vi "Drive Action.vi"(8 "Motor Saftey":T1, 11 "Operation States":T3) -> ()   [LabVIEW 2014]
uses:
  <vilib>/Rock Robotics/WPI/Solenoid/WPI_SolenoidValue.ctl
  <vilib>/Rock Robotics/WPI/SafetyOutput/WPI_SafetyOutputConfigMenu.ctl
  <vilib>/Rock Robotics/WPI/RobotDrive/WPI_RobotDriveGetSetRefNum.vi
  Robot Global Data.vi
  <vilib>/Rock Robotics/Network Tables/SD Write Numeric Array.vi
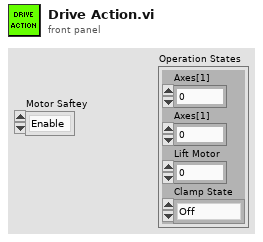
[diagram p1: front panel]
types:
  T1 = typedef "WPI_SafetyOutputConfigMenu.ctl" = enum16{"Enable", "Disable"}
  T2 = typedef "WPI_SolenoidValue.ctl" = enum16{"Off", "On", "Forward", "Reverse"}
  T3 = cluster{"Axes[1]":dbl, "Axes[1]":dbl, "Lift Motor":dbl, "Clamp State":T2}
  T4 = typedef "WPI_RobotDriveDevRef.ctl" = cluster{"DevStatus":errorcluster, "Motors[]":T5[], "Square Inputs":bool, "Max Output":dbl}
  T5 = typedef "WPI_MotorControlDeviceRef.ctl" = cluster{"DeviceStatus":errorcluster, "Type":T6, "PWM":cluster{"Controller":T7, "PWM Channel":T8, "DeadBand":T9}, "CAN":cluster{"Device Number":u8, "Control Mode":T10, "Semaphore":T11, "Max Vout":dbl, "TalonSRX Control Mode":T12}, "Invert":bool, "TransformRef":T13, "InvTransformRef":T13}
  T6 = typedef "WPI_MotorControlType.ctl" = enum16{"PWM", "CAN", "CANTalonSRX"}
  T7 = typedef "FPGA_TypedefDigitalModule.ctl" = enum16{"Controller 1"}
  T8 = typedef "FPGA_DIOPWMChannel.ctl" = enum8{"PWM 0", "PWM 1", "PWM 2", "PWM 3", "PWM 4", "PWM 5", "PWM 6", "PWM 7", "PWM 8", "PWM 9", "PWM MXP 0", "PWM MXP 1", "PWM MXP 2", "PWM MXP 3", "PWM MXP 4", "PWM MXP 5", "PWM MXP 6", "PWM MXP 7", "PWM MXP 8", "PWM MXP 9", "Invalid"}
  T9 = typedef "WPI_PWMDeadband.ctl" = cluster{"Name":string, "maxPositivePwm":i32, "minPositivePwm":i32, "centerPwm":i32, "maxNegativePwm":i32, "minNegativePwm":i32, "angularRange":u16}
  T10 = typedef "WPI_CANJaguar_ControlMode.ctl" = enum8{"Percent VBus", "Current", "Speed", "Position", "Voltage"}
  T11 = typedef "Semaphore RefNum" = refnum<k1>
  T12 = typedef "WPI_CANTalonSRX_APIControlMode.ctl" = enum8{"Percent VBus", "Speed", "Position", "Slave", "Unchanged / Invalid"}
  T13 = typedef "WPI_PWMTransform_ConPane.ctl" = refnum<vi>
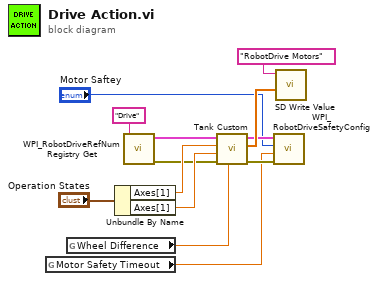
[diagram p0: block diagram]
diagram:
  n1 = global read "Robot Global Data.vi" "Motor Safety Timeout"() -> (w2:dbl)
  n2 = global read "Robot Global Data.vi" "Wheel Difference"() -> (w6:dbl)
  n3 = Unbundle By Name("Operation States") -> ("Axes[1]"=w9:dbl, "Axes[1]"=w8:dbl)
  n4 = call <vilib>:"WPI_RobotDriveRefNum Registry Get.vi"("refnum name"="Drive") -> ("error out"=w5:errorcluster, "RobotDriveDevRef"=w11:T4)  [unwired: 1 in, 8 out]
  n5 = call "Tank Custom.vi"("Wheel Difference"=w6, "error in (no error)"=w5, "Right axis value"=w8, "Left axis value"=w9, "RobotDriveDevRef"=w11) -> ("error out"=w4:errorcluster, "Motor Values"=w7:dbl[], "RobotDriveDevRef"=w3:T4)  [unwired: 4 in]
  n6 = call <vilib>:"WPI_RobotDriveSafetyConfig.vi"("error in (no error)"=w4, "timeout (s)"=w2, "mode"="Motor Saftey", "RobotDriveDevRef"=w3) -> ()  [unwired: 6 in, 2 out]
  n7 = call-poly <vilib>:"SD Write Value.vi"("Numeric Array"=w7, "Name"="RobotDrive Motors") -> ()  [unwired: 8 in, 2 out]
